vi "Update Data.vi"(8 "error in":errorcluster, 10 "Data":cluster{"Numeric":i32}, 11 "CutomOOB_Rx in":refnum<class "CIFTCustomOOB_Rx.lvclass">) -> (0 "error out":errorcluster, 3 "CutomOOB_Rx out":refnum<class "CIFTCustomOOB_Rx.lvclass">)   [LabVIEW 2021, in "CIFTCustomOOB_Rx.lvclass"]
uses:
  CIFTCustomOOB_Rx.lvclass
  D:/dev/CIF-LVCore/src/CIFUtilities/CIFOutOfBand/CIFOutOfBand.lvclass
  CIFUtilities/CIFOutOfBand/CIFOutOfBand.lvclass/CIFOutOfBand.ctl
  Typedef/Payload.ctl
  Typedef/OOB Commands.ctl
  CIFUtilities/CIFOutOfBand/CIFOutOfBand.lvclass
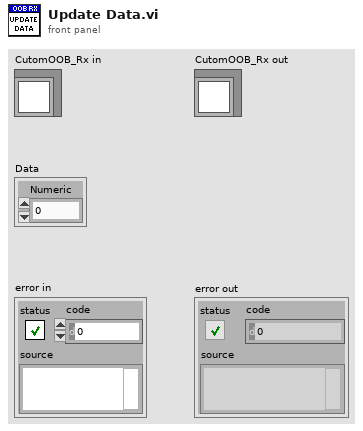
[diagram p1: front panel]
types:
  T1 = typedef "CIFTCustomOOB_Rx.lvclass/Payload.ctl" = cluster{"Data":cluster{"Numeric":i32}}
  T2 = typedef "CIFTCustomOOB_Rx.lvclass/OOB Commands.ctl" = enum8{"Update Data"}
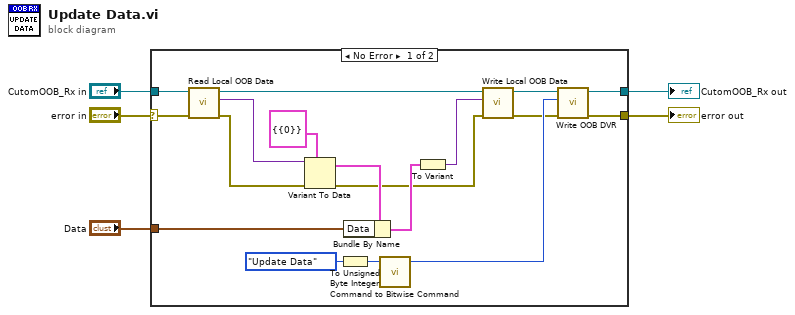
[diagram p0: block diagram]
diagram:
  n1 = case shown="No Error" "error in" {
    selector: "error in" -> [w7 w25]
    tunnel: [w22 w25] -> w4
    tunnel: "CutomOOB_Rx in" -> [w10 w24]
    tunnel: [w23 w24] -> w2
    tunnel: "Data" -> [w8 _]
    frame No Error {
      n2 = call "Read Local OOB Data.vi"("error in"=w7, "OOB in"=w10) -> ("error out"=w14:errorcluster, "Local OOB Data"=w17:variant, "OOB out"=w18:refnum<class "CIFTCustomOOB_Rx.lvclass">)  [unwired: 7 in]
      n3 = Variant To Data(error in=w14, type=T1 {"Data"={"Numeric"=0}} ("Template Payload"), Variant=w17) -> (data=w15:T1, error out=w11:errorcluster)
      n4 = To Unsigned Byte Integer(number=OOB_Commands."Update Data" ("OOB Main Commands")) -> (unsigned 8bit integer=w21:u8)
      n5 = Bundle By Name(cluster=w15, "Data"=w8) -> (w13:T1)
      n6 = call "Command to Bitwise Command.vi"("OOB Command"=w21) -> ("bit command"=w20:u64)  [unwired: 3 in]
      n7 = To Variant(anything=w13) -> (Variant=w12:variant)
      n8 = call "Write Local OOB Data.vi"("error in"=w11, "Local OOB Data"=w12, "OOB in"=w18) -> ("error out"=w6:errorcluster, "OOB out"=w9:refnum<class "CIFTCustomOOB_Rx.lvclass">)  [unwired: 7 in]
      n9 = call "Write OOB DVR.vi"("error in"=w6, "Commands (bitwise)"=w20, "OOB in"=w9) -> ("error out"=w22:errorcluster, "OOB out"=w23:refnum<class "CIFTCustomOOB_Rx.lvclass">)  [unwired: 7 in]
    }
    frame Error {
    }
  }
  "error out" <- w4
  "CutomOOB_Rx out" <- w2
